vi "FlexRIO-DMA-PROCESSING.vi"(5 "DMATtoHOSTFIFO":refnum<k21>="DMATtoHOST0", 6 "Base Clock":refnum<k21>, 7 "CHBUFFERS":T1={"CH0BUFFER"="FIFO0", "CH1BUFFER"="FIFO0", "CH2BUFFER"="FIFO0", "CH3BUFFER"="FIFO0"}, 8 "Enable":bool, 9 "NumberOfChannels":T2, 10 "DMA number":i32, 11 "DMA Control":T4={"DMATtoHOSTNCh"=[4], "DMATtoHOSTFrameType"=[0], "DMATtoHOSTSampleSize"=[2], "DMATtoHOSTBlockNWords"=[4096]}) -> ()   [LabVIEW 2013, in "IRIO.lvlib"]
uses:
  IRIO.lvlib
  ctl/DMAConfigParams.ctl
  ctl/NumberOfChannels.ctl
  ctl/AcquisitionStateControl.ctl
  <vilib>/Platform/TimedLoop/XDataNode/timing_clust.ctl
  <vilib>/Platform/TimedLoop/XDataNode/nitl_modes.ctl
  <vilib>/Platform/TimedLoop/XDataNode/wakeup.ctl
  <vilib>/rvi/Emulation/niFpgaSctlEmulationGetInTimedLoop.vi
  <vilib>/rvi/Emulation/niFpgaEmulationReportErrorSimple.vi
  <vilib>/rvi/Emulation/niFpgaGetClockAttributes.vi
  <vilib>/rvi/Emulation/niFpgaCriticalErrorInLSC.vi
  common/GlobalReg.vi
  <vilib>/rvi/DataTransferAndStorage/Container/Common/niFpgaContainerExecOnDevCompGetState.vi
  <vilib>/rvi/FIFO/Fifo_Resource/nirvififoEmulationGetNumberOfElementsToReadFpgaImpl.vi
  <vilib>/rvi/DataTransferAndStorage/Container/Common/niFpgaContainerGetUniqueNameForEmu.vi
  <vilib>/rvi/interface/RandomDataEmulation/nirviRandomDataFPGAFIFO.vi
  <vilib>/rvi/interface/RandomDataEmulation/niFpgaRandomDataHandleErrors.vi
  <vilib>/rvi/eio/common/nirviEmuReportErrorAndStop.vi
  <vilib>/rvi/FIFO/Fifo_Resource/nirvififoEmulationReadFpgaImpl.vi
  <vilib>/rvi/DataTransferAndStorage/Container/Common/niFpgaContainerSetEmuInfo.vi
  <vilib>/rvi/DataTransferAndStorage/Register/Emulation/niFpgaRegisterEmulationFpgaImpl.vi
  <instcachedir>/0/niFpgaRegisterEmulationFpgaImpl_DCF4BC0110594B98B44A971D60CEEC4D.lvgen/niFpgaRegisterEmulationFpgaImpl_DCF4BC0110594B98B44A971D60CEEC4D_003.vi
  <instcachedir>/0/niFpgaRegisterEmulationFpgaImpl_DCF4BC0110594B98B44A971D60CEEC4D.lvgen/niFpgaRegisterEmulationFpgaImpl_DCF4BC0110594B98B44A971D60CEEC4D_004.vi
  <vilib>/rvi/FIFO/Fifo_Resource/nirvififoEmulationWriteFpgaImpl.vi
  <vilib>/Platform/TimedLoop/XDataNode/XDataNode.xnode
  <vilib>/rvi/DataTransferAndStorage/Container/XNode/niFpgaContainer.xnode
  <vilib>/rvi/FIFO/Fifo_Resource/niFpgaFifoEmulationRefIn.vi
  <vilib>/rvi/LocalResourceManager/LocalResourceManager.xnode
  <vilib>/rvi/DataTransferAndStorage/Register/Emulation/niFpgaRegisterEmulationRefIn.vi
  <vilib>/Platform/TimedLoop/XDataNode/XDNodeRunTimeDep.lvlib
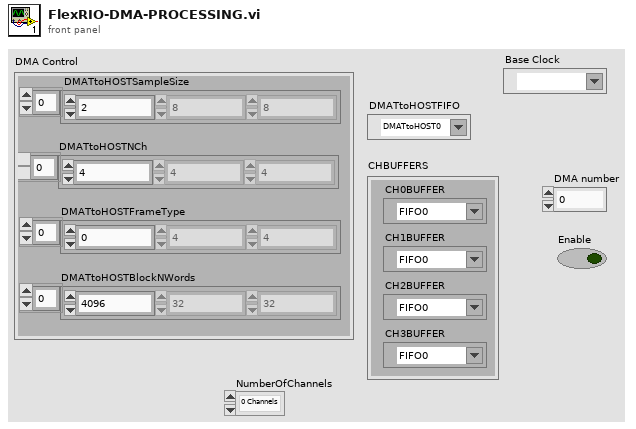
[diagram p1: front panel]
types:
  T1 = cluster{"CH0BUFFER":refnum<k21>, "CH1BUFFER":refnum<k21>, "CH2BUFFER":refnum<k21>, "CH3BUFFER":refnum<k21>}
  T2 = typedef "IRIO.lvlib/NumberOfChannels.ctl" = enum16{"0 Channels", "1 Channels", "2 Channels", "3 Channels", "4 Channels", "5 Channels", "6 Channels", "7 Channels", "8 Channels", "9 Channels", "10 Channels", "11 Channels", "12 Channels"}
  T3 = typedef "IRIO.lvlib/DMAConfigParams.ctl" = u16
  T4 = cluster{"DMATtoHOSTNCh":T3[], "DMATtoHOSTFrameType":u8[], "DMATtoHOSTSampleSize":u8[], "DMATtoHOSTBlockNWords":u16[]}
  T5 = typedef "IRIO.lvlib/AcquisitionStateControl.ctl" = enum16{"Idle", "Acq"}
  T6 = typedef "XDNodeRunTimeDep.lvlib/timing_clust.ctl" = cluster{"Expected End [f-1]":u64, "Actual End [f-1]":u64, "Finished Late? [f-1]":bool, "Expected End [i-1]":u64, "Actual End [i-1]":u64, "Finished Late? [i-1]":bool, "Expected Start [i]":u64, "Actual Start [i]":u64, "Expected Start [f]":u64, "Actual Start [f]":u64, "Source Name":string, "Structure Name":string, "Period":i64, "Deadline":i64, "Offset":i64, "Start":i64, "Priority":i32, "Timeout":i32, "Mode":T7, "Wakeup Reason":T8, "Error":errorcluster, "Source Type":string, "Secondary Source Type":string, "Global End Time":u64, "Global Start Time":u64, "Frame Duration":u64, "Iteration Duration":u64, "Assigned CPU":i32, "I/O Scan Engine Mode":u32}
  T7 = typedef "XDNodeRunTimeDep.lvlib/nitl_modes.ctl" = enum32{"No Change", "Process missed periods, maintain original phase", "Discard missed periods, maintain original phase", "Process missed periods, ignore original phase", "Discard missed periods, ignore original phase"}
  T8 = typedef "XDNodeRunTimeDep.lvlib/wakeup.ctl" = enum32{"Normal", "Aborted", "Asynchronous wakeup", "Timing source error", "Timed loop error", "Timeout"}
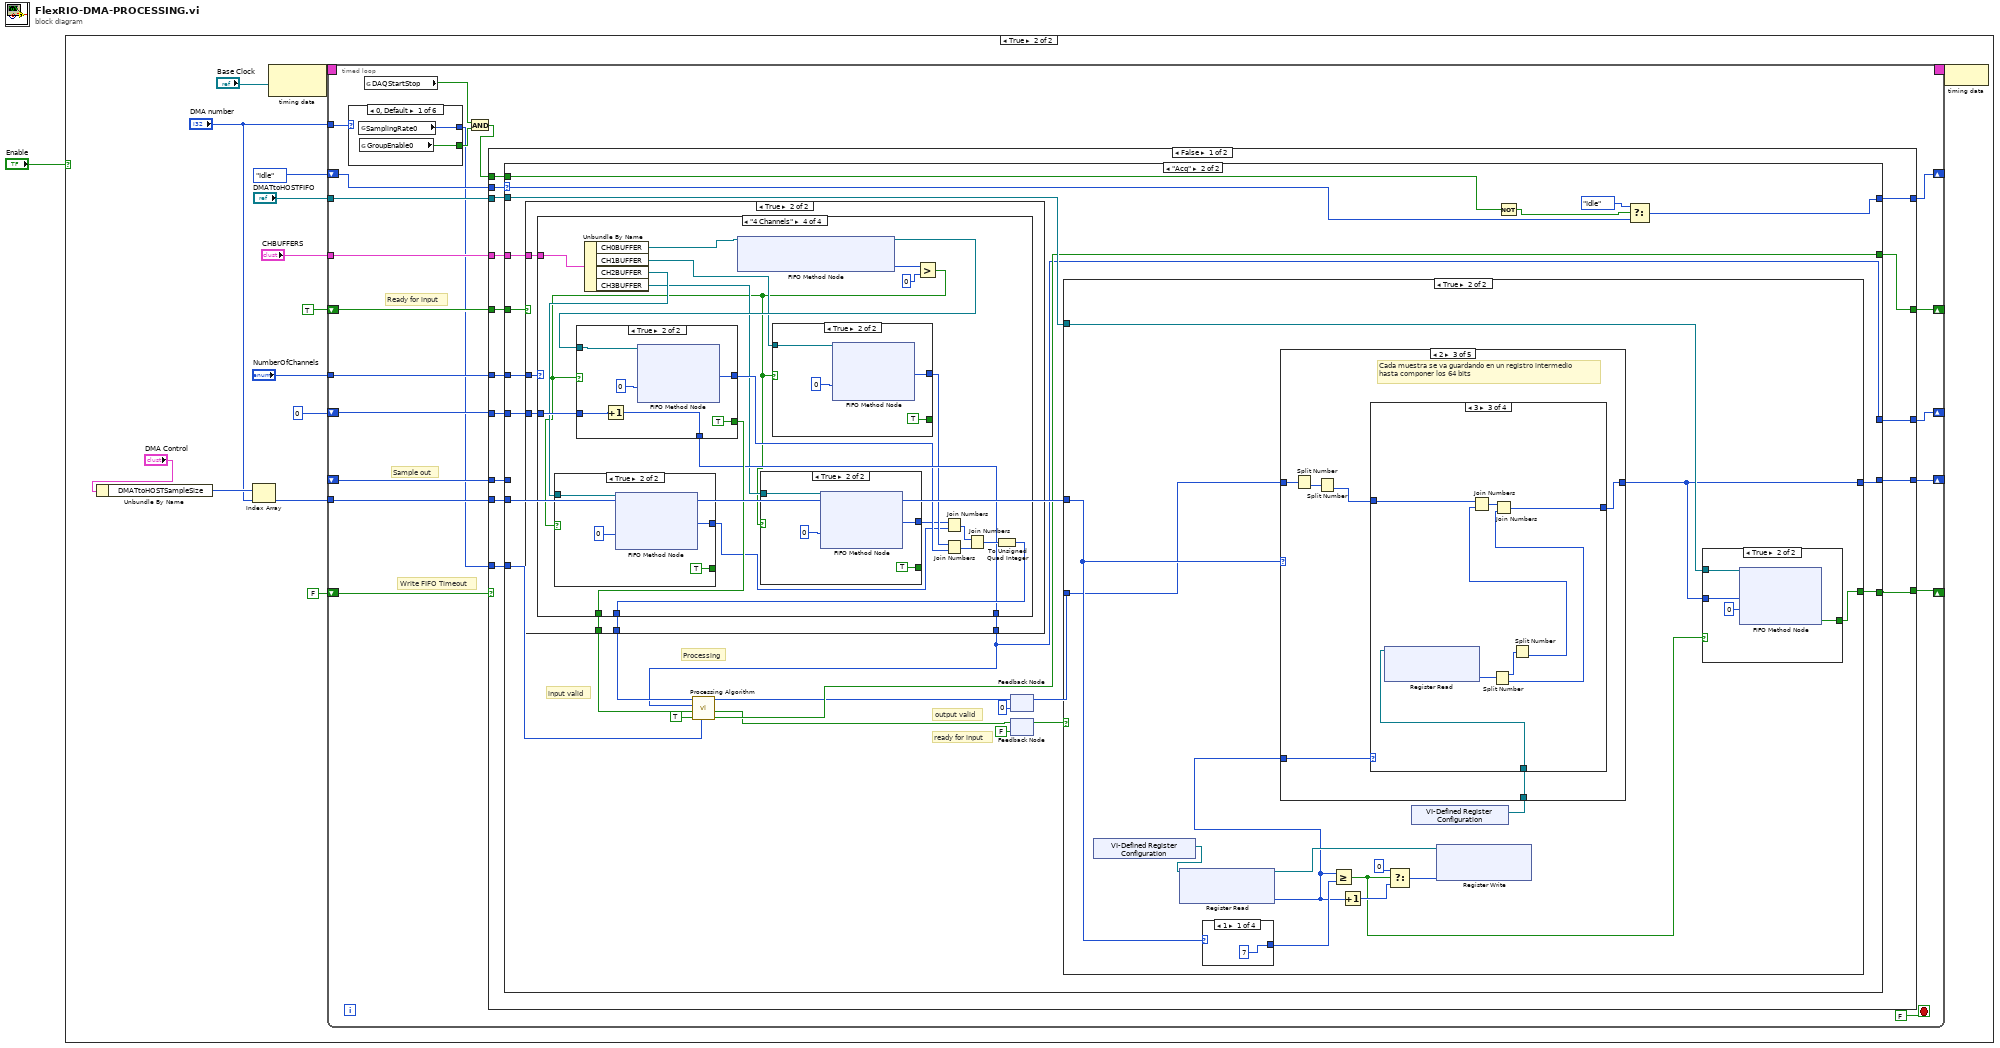
[diagram p0: block diagram]
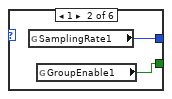
[diagram p3: hidden frame]
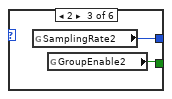
[diagram p4: hidden frame]
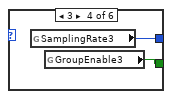
[diagram p5: hidden frame]
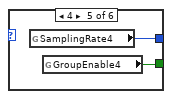
[diagram p6: hidden frame]
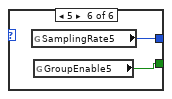
[diagram p7: hidden frame]
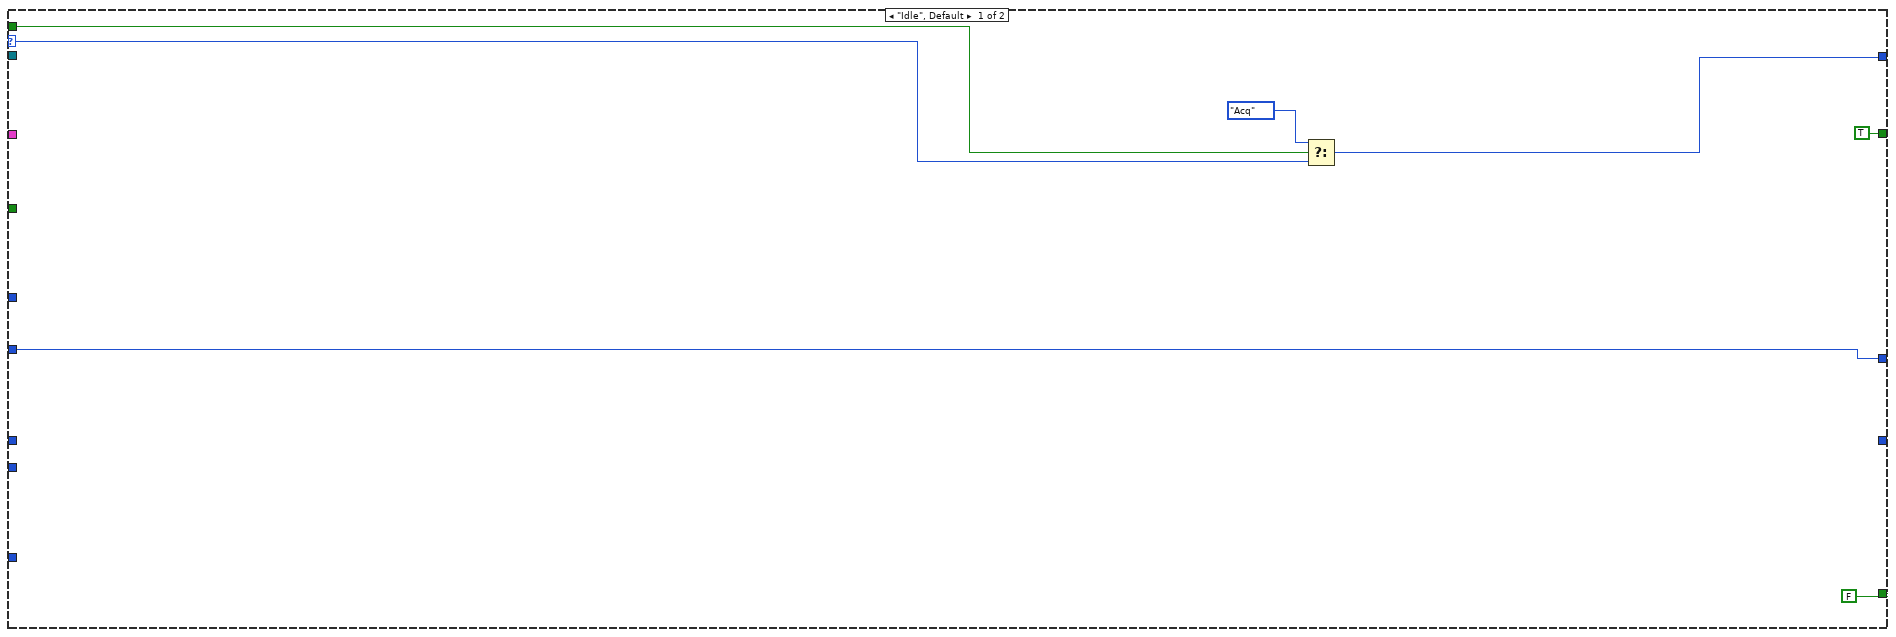
[diagram p8: hidden frame]
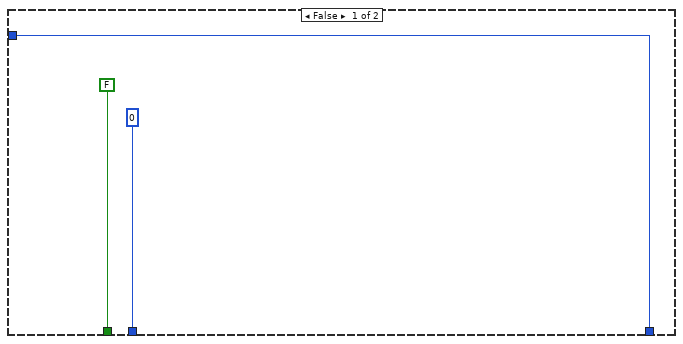
[diagram p9: hidden frame]
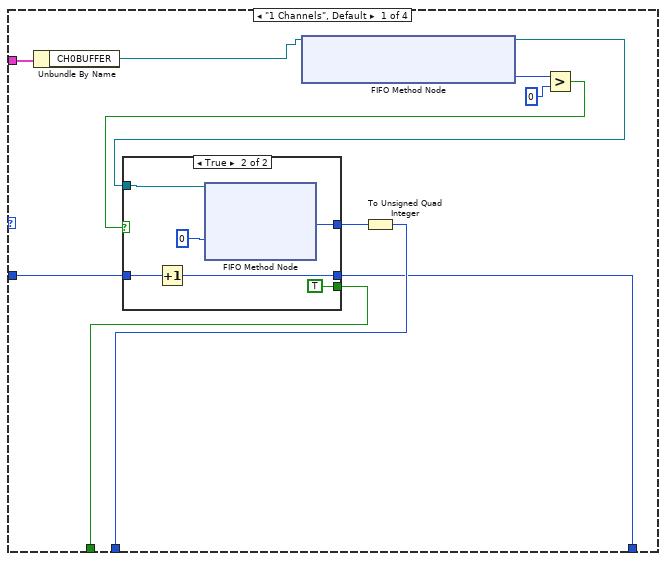
[diagram p10: hidden frame]
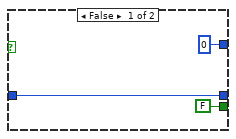
[diagram p11: hidden frame]
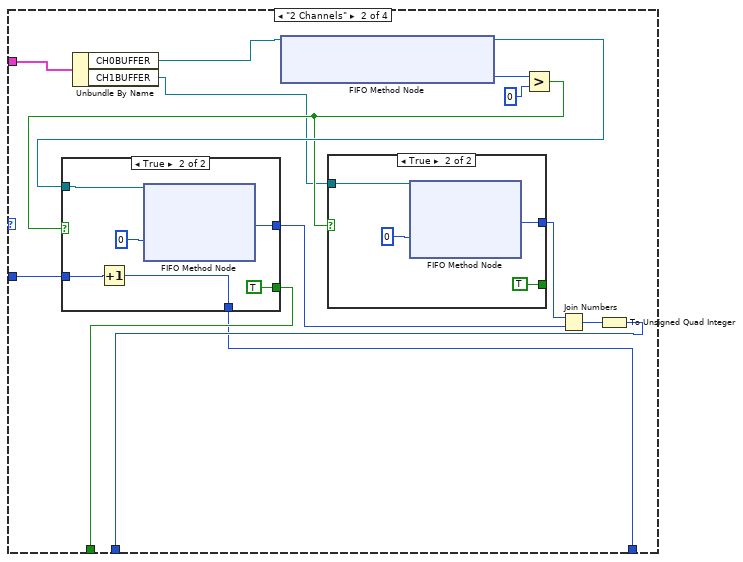
[diagram p12: hidden frame]
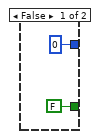
[diagram p13: hidden frame]
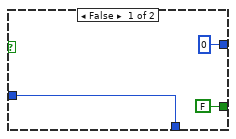
[diagram p14: hidden frame]
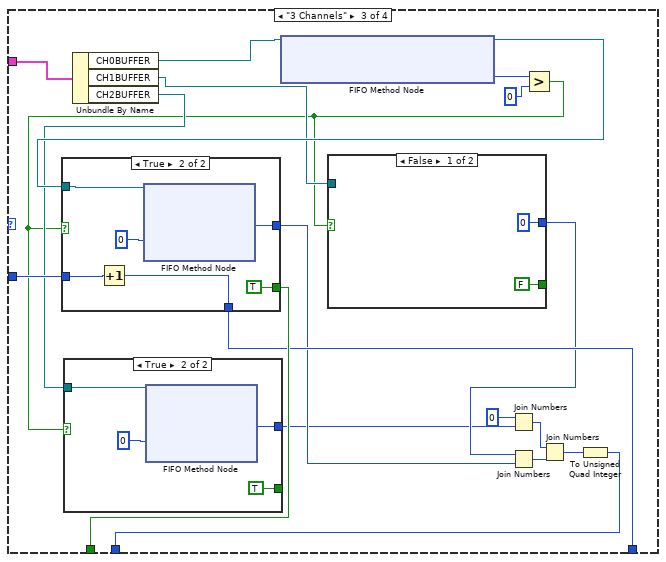
[diagram p15: hidden frame]
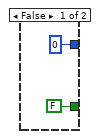
[diagram p16: hidden frame]
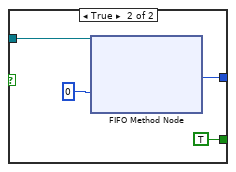
[diagram p17: hidden frame]
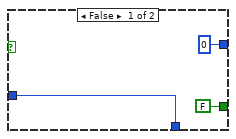
[diagram p18: hidden frame]
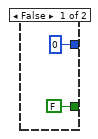
[diagram p19: hidden frame]
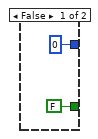
[diagram p20: hidden frame]
diagram:
  n1 = case shown="True" "Enable" {
    frame False {
    }
    frame True {
      n2 = Unbundle By Name("DMA Control") -> ("DMATtoHOSTSampleSize"=w14:u8[])
      n3 = Index Array(array=w14, index="DMA number") -> (element=w9:u8)
      n4 = node-c288("Base Clock") -> (w8:T6)
      n5 = timed-loop {
        shift-right: [w35] -> _
        shift-left: FALSE ("Timed Out?") -> [w34]
        shift-right: [w32] -> _
        shift-left: AcquisitionStateControl."Idle" ("Enum") -> [w33]
        tunnel: "DMATtoHOSTFIFO" -> [w31]
        shift-right: [w30] -> _
        shift-left: _ -> [w29]
        tunnel: "DMA number" -> [w28]
        tunnel: w9 -> [w24]
        timing: w8 -> [_]
        timing-out: [_] -> w7
        shift-right: [w21] -> _
        shift-left: TRUE ("ready for input") -> [w22]
        tunnel: "NumberOfChannels" -> [w20]
        tunnel: "CHBUFFERS" -> [w19]
        shift-right: [w18] -> _
        shift-left: u64 0 -> [w17]
        stop <- FALSE stop-if-true
        # "Sample out"
        # "Write FIFO Timeout"
        # "Ready for input"
        n6 = case shown="0, Default" w28 {
          tunnel: [w37 w39 w41 w43 w45 w47] -> w16
          tunnel: [w36 w38 w40 w42 w44 w46] -> w26
          frame 0, Default {
            n7 = global read "GlobalReg.vi" "SamplingRate0"() -> (w37:u16)
            n8 = global read "GlobalReg.vi" "GroupEnable0"() -> (w36:bool)
          }
          frame 1 {
            n9 = global read "GlobalReg.vi" "SamplingRate1"() -> (w39:u16)
            n10 = global read "GlobalReg.vi" "GroupEnable1"() -> (w38:bool)
          }
          frame 2 {
            n11 = global read "GlobalReg.vi" "SamplingRate2"() -> (w41:u16)
            n12 = global read "GlobalReg.vi" "GroupEnable2"() -> (w40:bool)
          }
          frame 3 {
            n13 = global read "GlobalReg.vi" "SamplingRate3"() -> (w43:u16)
            n14 = global read "GlobalReg.vi" "GroupEnable3"() -> (w42:bool)
          }
          frame 4 {
            n15 = global read "GlobalReg.vi" "SamplingRate4"() -> (w45:u16)
            n16 = global read "GlobalReg.vi" "GroupEnable4"() -> (w44:bool)
          }
          frame 5 {
            n17 = global read "GlobalReg.vi" "SamplingRate5"() -> (w47:u16)
            n18 = global read "GlobalReg.vi" "GroupEnable5"() -> (w46:bool)
          }
        }
        n19 = global read "GlobalReg.vi" "DAQStartStop"() -> (w25:bool)
        n20 = And(x=w25, y=w26) -> (x .and. y?=w27:bool)
        n21 = case shown="False" w34 {
          tunnel: [w57 w404] -> w35
          tunnel: w33 -> [w62 w407]
          tunnel: [w61 w407] -> w32
          tunnel: w31 -> [w60 w406]
          tunnel: [w59 w405] -> w30
          tunnel: w29 -> [w58 w405]
          tunnel: w27 -> [w56 _]
          tunnel: w24 -> [w55 _]
          tunnel: w22 -> [w54 w403]
          tunnel: [w53 w403] -> w21
          tunnel: w20 -> [w52 _]
          tunnel: w19 -> [w51 _]
          tunnel: w17 -> [w50 w402]
          tunnel: [w49 w402] -> w18
          tunnel: w16 -> [w48 _]
          frame False {
            n22 = case shown="\"Acq\"" w62 {
              selector: w62 -> [w68 w93]
              tunnel: [w67 w92] -> w61
              tunnel: w60 -> [_ w85]
              tunnel: [_ w90] -> w59
              tunnel: w58 -> [_ _]
              tunnel: [FALSE ("Timed Out?") w89] -> w57
              tunnel: w56 -> [w65 w88]
              tunnel: w55 -> [_ w84]
              tunnel: w54 -> [_ w76]
              tunnel: [TRUE ("ready for input") w83] -> w53
              tunnel: w52 -> [_ w74]
              tunnel: w51 -> [_ w73]
              tunnel: w50 -> [w63 w72]
              tunnel: [w63 w70] -> w49
              tunnel: w48 -> [_ w71]
              frame "Idle", Default {
                n23 = Select(t=AcquisitionStateControl."Acq" ("Enum"), s=w65, f=w68) -> (s? t:f=w67:T5)
              }
              frame "Acq" {
                # "output valid"
                # "ready for input"
                # "input valid"
                # "Processing"
                n24 = case shown="True" w76 {
                  tunnel: [u64 0 ("Element") w103] -> w87
                  tunnel: [FALSE w102] -> w86
                  tunnel: w74 -> [_ w101]
                  tunnel: w73 -> [_ w100]
                  tunnel: w72 -> [w95 w99]
                  tunnel: [w95 w98] -> w70
                  frame False {
                  }
                  frame True {
                    n25 = case shown="\"4 Channels\"" w101 {
                      tunnel: [w108 w130 w166 w207] -> w103
                      tunnel: [w110 w134 w168 w209] -> w102
                      tunnel: w100 -> [w107 w128 w165 w206]
                      tunnel: w99 -> [w105 w125 w162 w203]
                      tunnel: [w104 w124 w161 w202] -> w98
                      frame "1 Channels", Default {
                        n26 = Unbundle By Name(w107) -> ("CH0BUFFER"=w106:refnum<k21>)
                        n27 = xnode ("FIFO Method Node")("FIFO In"=w106) -> ("Number of Elements to Read"=w113:u32, "FIFO Out"=w114:refnum<k21>)
                        n28 = Greater?(x=w113, y=u32 0) -> (0:w111:bool)
                        n29 = case shown="True" w111 {
                          tunnel: w114 -> [_ w122]
                          tunnel: [i16 0 ("Element") w121] -> w109
                          tunnel: [FALSE TRUE] -> w110
                          tunnel: w105 -> [w115 w119]
                          tunnel: [w115 w118] -> w104
                          frame False {
                          }
                          frame True {
                            n30 = Increment(x=w119) -> (x+1=w118:u64)
                            n31 = xnode ("FIFO Method Node")("Timeout"=0, "FIFO In"=w122) -> ("Element"=w121:i16)  [unwired: 2 out]
                          }
                        }
                        n32 = To Unsigned Quad Integer(1:w109) -> (0:w108:u64)
                      }
                      frame "2 Channels" {
                        n33 = Unbundle By Name(w128) -> ("CH0BUFFER"=w127:refnum<k21>, "CH1BUFFER"=w126:refnum<k21>)
                        n34 = xnode ("FIFO Method Node")("FIFO In"=w127) -> ("Number of Elements to Read"=w136:u32, "FIFO Out"=w137:refnum<k21>)
                        n35 = Greater?(x=w136, y=u32 0) -> (0:w129:bool)
                        n36 = case shown="True" w129 {
                          tunnel: w137 -> [_ w151]
                          tunnel: [i16 0 ("Element") w150] -> w132
                          tunnel: [FALSE TRUE] -> w134
                          tunnel: w125 -> [w144 w148]
                          tunnel: [w144 w147] -> w124
                          frame False {
                          }
                          frame True {
                            n37 = Increment(x=w148) -> (x+1=w147:u64)
                            n38 = xnode ("FIFO Method Node")("Timeout"=0, "FIFO In"=w151) -> ("Element"=w150:i16)  [unwired: 2 out]
                          }
                        }
                        n39 = case shown="True" w129 {
                          tunnel: w126 -> [_ w140]
                          tunnel: [i16 0 ("Element") w142] -> w133
                          tunnel: [FALSE TRUE] -> _
                          frame False {
                          }
                          frame True {
                            n40 = xnode ("FIFO Method Node")("Timeout"=0, "FIFO In"=w140) -> ("Element"=w142:i16)  [unwired: 2 out]
                          }
                        }
                        n41 = Join Numbers(hi=w133, lo=w132) -> ((hi.lo)=w131:u32)
                        n42 = To Unsigned Quad Integer(1:w131) -> (0:w130:u64)
                      }
                      frame "3 Channels" {
                        n43 = Unbundle By Name(w165) -> ("CH0BUFFER"=w164:refnum<k21>, "CH1BUFFER"=w163:refnum<k21>, "CH2BUFFER"=w160:refnum<k21>)
                        n44 = xnode ("FIFO Method Node")("FIFO In"=w164) -> ("Number of Elements to Read"=w170:u32, "FIFO Out"=w171:refnum<k21>)
                        n45 = Greater?(x=w170, y=u32 0) -> (0:w153:bool)
                        n46 = case shown="True" w153 {
                          tunnel: w171 -> [_ w191]
                          tunnel: [i16 0 ("Element") w190] -> w159
                          tunnel: [FALSE TRUE] -> w168
                          tunnel: w162 -> [w184 w188]
                          tunnel: [w184 w187] -> w161
                          frame False {
                          }
                          frame True {
                            n47 = Increment(x=w188) -> (x+1=w187:u64)
                            n48 = xnode ("FIFO Method Node")("Timeout"=0, "FIFO In"=w191) -> ("Element"=w190:i16)  [unwired: 2 out]
                          }
                        }
                        n49 = case shown="True" w153 {
                          tunnel: w160 -> [_ w174]
                          tunnel: [i16 0 ("Element") w176] -> w155
                          tunnel: [FALSE TRUE] -> _
                          frame False {
                          }
                          frame True {
                            n50 = xnode ("FIFO Method Node")("Timeout"=0, "FIFO In"=w174) -> ("Element"=w176:i16)  [unwired: 2 out]
                          }
                        }
                        n51 = case shown="False" w153 {
                          tunnel: w163 -> [_ w180]
                          tunnel: [i16 0 ("Element") w182] -> w158
                          tunnel: [FALSE TRUE] -> _
                          frame False {
                          }
                          frame True {
                            n52 = xnode ("FIFO Method Node")("Timeout"=0, "FIFO In"=w180) -> ("Element"=w182:i16)  [unwired: 2 out]
                          }
                        }
                        n53 = Join Numbers(hi=i16 0, lo=w155) -> ((hi.lo)=w156:u32)
                        n54 = Join Numbers(hi=w158, lo=w159) -> ((hi.lo)=w157:u32)
                        n55 = Join Numbers(hi=w156, lo=w157) -> ((hi.lo)=w167:u64)
                        n56 = To Unsigned Quad Integer(1:w167) -> (0:w166:u64)
                      }
                      frame "4 Channels" {
                        n57 = Unbundle By Name(w206) -> ("CH0BUFFER"=w205:refnum<k21>, "CH1BUFFER"=w204:refnum<k21>, "CH2BUFFER"=w201:refnum<k21>, "CH3BUFFER"=w195:refnum<k21>)
                        n58 = xnode ("FIFO Method Node")("FIFO In"=w205) -> ("Number of Elements to Read"=w211:u32, "FIFO Out"=w212:refnum<k21>)
                        n59 = Greater?(x=w211, y=u32 0) -> (0:w193:bool)
                        n60 = case shown="True" w193 {
                          tunnel: w201 -> [_ w221]
                          tunnel: [i16 0 ("Element") w223] -> w196
                          tunnel: [FALSE TRUE] -> _
                          frame False {
                          }
                          frame True {
                            n61 = xnode ("FIFO Method Node")("Timeout"=0, "FIFO In"=w221) -> ("Element"=w223:i16)  [unwired: 2 out]
                          }
                        }
                        n62 = case shown="True" w193 {
                          tunnel: w212 -> [_ w238]
                          tunnel: [i16 0 ("Element") w237] -> w200
                          tunnel: [FALSE TRUE] -> w209
                          tunnel: w203 -> [w231 w235]
                          tunnel: [w231 w234] -> w202
                          frame False {
                          }
                          frame True {
                            n63 = Increment(x=w235) -> (x+1=w234:u64)
                            n64 = xnode ("FIFO Method Node")("Timeout"=0, "FIFO In"=w238) -> ("Element"=w237:i16)  [unwired: 2 out]
                          }
                        }
                        n65 = case shown="True" w193 {
                          tunnel: w195 -> [_ w215]
                          tunnel: [i16 0 ("Element") w217] -> w194
                          tunnel: [FALSE TRUE] -> _
                          frame False {
                          }
                          frame True {
                            n66 = xnode ("FIFO Method Node")("Timeout"=0, "FIFO In"=w215) -> ("Element"=w217:i16)  [unwired: 2 out]
                          }
                        }
                        n67 = case shown="True" w193 {
                          tunnel: w204 -> [_ w227]
                          tunnel: [i16 0 ("Element") w229] -> w199
                          tunnel: [FALSE TRUE] -> _
                          frame False {
                          }
                          frame True {
                            n68 = xnode ("FIFO Method Node")("Timeout"=0, "FIFO In"=w227) -> ("Element"=w229:i16)  [unwired: 2 out]
                          }
                        }
                        n69 = Join Numbers(hi=w194, lo=w196) -> ((hi.lo)=w197:u32)
                        n70 = Join Numbers(hi=w199, lo=w200) -> ((hi.lo)=w198:u32)
                        n71 = Join Numbers(hi=w197, lo=w198) -> ((hi.lo)=w208:u64)
                        n72 = To Unsigned Quad Integer(1:w208) -> (0:w207:u64)
                      }
                    }
                  }
                }
                n73 = call "Processing Algorithm.vi"("Sampling Rate"=w71, "ready for output (T)"=TRUE, "input valid"=w86, "Sample Number"=w70, "Sample in"=w87) -> ("ready for input"=w83:bool, "output valid"=w82:bool, "Sample out"=w80:u64)  [unwired: 4 in]
                n74 = feedback #1(i64 0 ("Sample out")) -> (w79:u64)
                n75 = feedback-in #1(w80) -> ()
                n76 = feedback #2(FALSE ("output valid")) -> (w81:bool)
                n77 = feedback-in #2(w82) -> ()
                n78 = case shown="True" w81 {
                  tunnel: [FALSE ("Timed Out?") w247] -> w89
                  tunnel: [_ w245] -> w90
                  tunnel: w85 -> [_ w246]
                  tunnel: w84 -> [_ w242]
                  tunnel: w79 -> [_ w241]
                  frame False {
                  }
                  frame True {
                    n79 = xnode ("VI-Defined Register Configuration")() -> ("Register Out"=w254:refnum<k21>)
                    n80 = xnode ("Register Read")("Register In"=w254) -> ("Register Out"=w253:refnum<k21>, "Data"=w243:u8)
                    n81 = case shown="1" w242 {
                      tunnel: [u8 7 u8 3 u8 1 u8 0] -> w252
                      frame 1 {
                      }
                      frame 2 {
                      }
                      frame 4 {
                      }
                      frame 8, Default {
                      }
                    }
                    n82 = Greater Or Equal?(x=w243, y=w252) -> (x >= y?=w244:bool)
                    n83 = Increment(x=w243) -> (x+1=w249:u8)
                    n84 = Select(t=u8 0 ("f"), s=w244, f=w249) -> (s? t:f=w251:u8)
                    n85 = xnode ("VI-Defined Register Configuration")() -> ("Register Out"=w248:refnum<k21>)
                    n86 = case shown="2" w242 {
                      tunnel: w248 -> [_ w262 w349 w382 _]
                      tunnel: [u64 0 w261 w348 w381 w392] -> w245
                      tunnel: w241 -> [_ w260 w347 w380 w392]
                      tunnel: w243 -> [_ w256 w344 w378 _]
                      frame 0, Default {
                      }
                      frame 1 {
                        # "Cada muestra se va guardando en un registro intermedio\nhasta componer los 64 bits"
                        n87 = Split Number(x=w260) -> (lo(x)=w259:u32)  [unwired: 1 out]
                        n88 = Split Number(x=w259) -> (lo(x)=w258:u16)  [unwired: 1 out]
                        n89 = Split Number(x=w258) -> (lo(x)=w257:u8)  [unwired: 1 out]
                        n90 = case shown="6" w256 {
                          tunnel: [w266 w279 w290 w301 w312 w322 w331 w338] -> w261
                          tunnel: w262 -> [w272 w282 w293 w303 w314 w324 w330 w342]
                          tunnel: w257 -> [w264 w276 w286 w296 w305 w316 w327 w339]
                          frame 1 {
                            n91 = xnode ("Register Read")("Register In"=w272) -> ("Data"=w271:u64)  [unwired: 1 out]
                            n92 = Split Number(x=w271) -> (lo(x)=w273:u32)  [unwired: 1 out]
                            n93 = Split Number(x=w273) -> (lo(x)=w270:u16)  [unwired: 1 out]
                            n94 = Split Number(x=w270) -> (lo(x)=w265:u8)  [unwired: 1 out]
                            n95 = Join Numbers(hi=w264, lo=w265) -> ((hi.lo)=w269:u16)
                            n96 = Join Numbers(hi=u16 0, lo=w269) -> ((hi.lo)=w268:u32)
                            n97 = Join Numbers(hi=u32 0, lo=w268) -> ((hi.lo)=w266:u64)
                            n98 = xnode ("Register Write")("Data"=w266, "Register In"=w272) -> ()  [unwired: 1 out]
                          }
                          frame 2 {
                            n99 = xnode ("Register Read")("Register In"=w282) -> ("Data"=w281:u64)  [unwired: 1 out]
                            n100 = Join Numbers(hi=u8 0, lo=w276) -> ((hi.lo)=w278:u16)
                            n101 = Split Number(x=w281) -> (lo(x)=w283:u32)  [unwired: 1 out]
                            n102 = Split Number(x=w283) -> (lo(x)=w275:u16)  [unwired: 1 out]
                            n103 = Join Numbers(hi=w278, lo=w275) -> ((hi.lo)=w280:u32)
                            n104 = Join Numbers(hi=u32 0, lo=w280) -> ((hi.lo)=w279:u64)
                            n105 = xnode ("Register Write")("Data"=w279, "Register In"=w282) -> ()  [unwired: 1 out]
                          }
                          frame 3 {
                            n106 = xnode ("Register Read")("Register In"=w293) -> ("Data"=w292:u64)  [unwired: 1 out]
                            n107 = Split Number(x=w292) -> (lo(x)=w294:u32)  [unwired: 1 out]
                            n108 = Split Number(x=w294) -> (hi(x)=w287:u16, lo(x)=w285:u16)
                            n109 = Split Number(x=w287) -> (lo(x)=w284:u8)  [unwired: 1 out]
                            n110 = Join Numbers(hi=w286, lo=w284) -> ((hi.lo)=w289:u16)
                            n111 = Join Numbers(hi=w289, lo=w285) -> ((hi.lo)=w291:u32)
                            n112 = Join Numbers(hi=u32 0, lo=w291) -> ((hi.lo)=w290:u64)
                            n113 = xnode ("Register Write")("Data"=w290, "Register In"=w293) -> ()  [unwired: 1 out]
                          }
                          frame 4 {
                            n114 = xnode ("Register Read")("Register In"=w303) -> ("Data"=w302:u64)  [unwired: 1 out]
                            n115 = Join Numbers(hi=u8 0, lo=w296) -> ((hi.lo)=w298:u16)
                            n116 = Join Numbers(hi=u16 0, lo=w298) -> ((hi.lo)=w299:u32)
                            n117 = Split Number(x=w302) -> (lo(x)=w300:u32)  [unwired: 1 out]
                            n118 = Join Numbers(hi=w299, lo=w300) -> ((hi.lo)=w301:u64)
                            n119 = xnode ("Register Write")("Data"=w301, "Register In"=w303) -> ()  [unwired: 1 out]
                          }
                          frame 5 {
                            n120 = xnode ("Register Read")("Register In"=w314) -> ("Data"=w313:u64)  [unwired: 1 out]
                            n121 = Split Number(x=w313) -> (hi(x)=w307:u32, lo(x)=w311:u32)
                            n122 = Split Number(x=w307) -> (lo(x)=w306:u16)  [unwired: 1 out]
                            n123 = Split Number(x=w306) -> (lo(x)=w304:u8)  [unwired: 1 out]
                            n124 = Join Numbers(hi=w305, lo=w304) -> ((hi.lo)=w309:u16)
                            n125 = Join Numbers(hi=u16 0, lo=w309) -> ((hi.lo)=w310:u32)
                            n126 = Join Numbers(hi=w310, lo=w311) -> ((hi.lo)=w312:u64)
                            n127 = xnode ("Register Write")("Data"=w312, "Register In"=w314) -> ()  [unwired: 1 out]
                          }
                          frame 6 {
                            n128 = xnode ("Register Read")("Register In"=w324) -> ("Data"=w323:u64)  [unwired: 1 out]
                            n129 = Join Numbers(hi=u8 0, lo=w316) -> ((hi.lo)=w318:u16)
                            n130 = Split Number(x=w323) -> (hi(x)=w319:u32, lo(x)=w321:u32)
                            n131 = Split Number(x=w319) -> (lo(x)=w317:u16)  [unwired: 1 out]
                            n132 = Join Numbers(hi=w318, lo=w317) -> ((hi.lo)=w320:u32)
                            n133 = Join Numbers(hi=w320, lo=w321) -> ((hi.lo)=w322:u64)
                            n134 = xnode ("Register Write")("Data"=w322, "Register In"=w324) -> ()  [unwired: 1 out]
                          }
                          frame 7 {
                            n135 = xnode ("Register Read")("Register In"=w330) -> ("Data"=w329:u64)  [unwired: 1 out]
                            n136 = Split Number(x=w329) -> (hi(x)=w333:u32, lo(x)=w335:u32)
                            n137 = Split Number(x=w333) -> (hi(x)=w326:u16, lo(x)=w332:u16)
                            n138 = Split Number(x=w326) -> (lo(x)=w325:u8)  [unwired: 1 out]
                            n139 = Join Numbers(hi=w327, lo=w325) -> ((hi.lo)=w328:u16)
                            n140 = Join Numbers(hi=w328, lo=w332) -> ((hi.lo)=w334:u32)
                            n141 = Join Numbers(hi=w334, lo=w335) -> ((hi.lo)=w331:u64)
                          }
                          frame 0, Default {
                            n142 = Join Numbers(hi=u8 0, lo=w339) -> ((hi.lo)=w343:u16)
                            n143 = Join Numbers(hi=u16 0, lo=w343) -> ((hi.lo)=w341:u32)
                            n144 = Join Numbers(hi=u32 0, lo=w341) -> ((hi.lo)=w338:u64)
                            n145 = xnode ("Register Write")("Data"=w338, "Register In"=w342) -> ()  [unwired: 1 out]
                          }
                        }
                      }
                      frame 2 {
                        # "Cada muestra se va guardando en un registro intermedio\nhasta componer los 64 bits"
                        n146 = Split Number(x=w347) -> (lo(x)=w346:u32)  [unwired: 1 out]
                        n147 = Split Number(x=w346) -> (lo(x)=w345:u16)  [unwired: 1 out]
                        n148 = case shown="3" w344 {
                          tunnel: [w353 w362 w368 w374] -> w348
                          tunnel: w349 -> [w356 w364 w367 w377]
                          tunnel: w345 -> [w350 w358 w365 w373]
                          frame 1 {
                            n149 = xnode ("Register Read")("Register In"=w356) -> ("Data"=w355:u64)  [unwired: 1 out]
                            n150 = Split Number(x=w355) -> (lo(x)=w357:u32)  [unwired: 1 out]
                            n151 = Split Number(x=w357) -> (lo(x)=w351:u16)  [unwired: 1 out]
                            n152 = Join Numbers(hi=w350, lo=w351) -> ((hi.lo)=w354:u32)
                            n153 = Join Numbers(hi=u16 0, lo=w354) -> ((hi.lo)=w353:u64)
                            n154 = xnode ("Register Write")("Data"=w353, "Register In"=w356) -> ()  [unwired: 1 out]
                          }
                          frame 2 {
                            n155 = xnode ("Register Read")("Register In"=w364) -> ("Data"=w363:u64)  [unwired: 1 out]
                            n156 = Join Numbers(hi=u16 0, lo=w358) -> ((hi.lo)=w360:u32)
                            n157 = Split Number(x=w363) -> (lo(x)=w361:u32)  [unwired: 1 out]
                            n158 = Join Numbers(hi=w360, lo=w361) -> ((hi.lo)=w362:u64)
                            n159 = xnode ("Register Write")("Data"=w362, "Register In"=w364) -> ()  [unwired: 1 out]
                          }
                          frame 3 {
                            n160 = xnode ("Register Read")("Register In"=w367) -> ("Data"=w366:u64)  [unwired: 1 out]
                            n161 = Split Number(x=w366) -> (hi(x)=w370:u32, lo(x)=w372:u32)
                            n162 = Split Number(x=w370) -> (lo(x)=w369:u16)  [unwired: 1 out]
                            n163 = Join Numbers(hi=w365, lo=w369) -> ((hi.lo)=w371:u32)
                            n164 = Join Numbers(hi=w371, lo=w372) -> ((hi.lo)=w368:u64)
                          }
                          frame 0, Default {
                            w375 = u16 0 ("hi")
                            n165 = Join Numbers(hi=w375, lo=w373) -> ((hi.lo)=w376:u32)
                            n166 = Join Numbers(hi=w375, lo=w376) -> ((hi.lo)=w374:u64)
                            n167 = xnode ("Register Write")("Data"=w374, "Register In"=w377) -> ()  [unwired: 1 out]
                          }
                        }
                      }
                      frame 4 {
                        # "Cada muestra se va guardando en un registro intermedio\nhasta componer los 64 bits"
                        n168 = Split Number(x=w380) -> (lo(x)=w379:u32)  [unwired: 1 out]
                        n169 = case shown="0, Default" w378 {
                          tunnel: [w386 w389] -> w381
                          tunnel: w382 -> [w385 w391]
                          tunnel: w379 -> [w383 w388]
                          frame 1 {
                            n170 = xnode ("Register Read")("Register In"=w385) -> ("Data"=w384:u64)  [unwired: 1 out]
                            n171 = Split Number(x=w384) -> (lo(x)=w387:u32)  [unwired: 1 out]
                            n172 = Join Numbers(hi=w383, lo=w387) -> ((hi.lo)=w386:u64)
                          }
                          frame 0, Default {
                            n173 = Join Numbers(hi=u16 0, lo=w388) -> ((hi.lo)=w389:u64)
                            n174 = xnode ("Register Write")("Data"=w389, "Register In"=w391) -> ()  [unwired: 1 out]
                          }
                        }
                      }
                      frame 8 {
                      }
                    }
                    n175 = xnode ("Register Write")("Data"=w251, "Register In"=w253) -> ()  [unwired: 1 out]
                    n176 = case shown="True" w244 {
                      tunnel: [FALSE ("Timed Out?") w396] -> w247
                      tunnel: w246 -> [_ w395]
                      tunnel: w245 -> [_ w394]
                      frame False {
                      }
                      frame True {
                        n177 = xnode ("FIFO Method Node")("Element"=w394, "Timeout"=0, "FIFO In"=w395) -> ("Timed Out?"=w396:bool)  [unwired: 1 out]
                      }
                    }
                  }
                }
                n178 = Not(x=w88) -> (.not. x?=w91:bool)
                n179 = Select(t=AcquisitionStateControl."Idle" ("Enum"), s=w91, f=w93) -> (s? t:f=w92:T5)
              }
            }
          }
          frame True {
            n180 = xnode ("FIFO Method Node")("Element"=w405, "Timeout"=0, "FIFO In"=w406) -> ("Timed Out?"=w404:bool)  [unwired: 1 out]
          }
        }
      }
      n181 = node-c288(w7) -> ()
    }
  }
